vi "Day 4 - Part two.vi"() -> ()   [LabVIEW 2023]
panel:
  out "appended array":string[][](array[string])
  out "sum":i16
  in  "input":string="71-89,66-70\n24-70,23-55\n19-85,18-86\n50-90,50-95\n55-55,56-72\n3-65,5-66\n98-99,66-99\n14-67,14-14\n4-79,78-79\n13-98,10-98\n27-78,77-78\n22-28,22-27\n84-99,98-99\n7-96,99-99\n33-54,34-54\n29-45,44-44\n18-48,57-78\n89-95,89-93\n39-53,63-99\n13-95,94-95\n7-43,7-42\n16-16,16-96\n41-68,68-87\n83-83,73-82\n65-95,64-71\n5-98,5-95\n51-54,50-99\n33-39,36-74\n9-73,10-86\n20-31,21-59\n12-27,11-12\n10-96,7-11\n55-71,70-77\n13-97,3-14\n5-99,5-5\n25-98,25-98\n81-94,81-94\n26-42,49-74\n77-98,31-77\n8-77,6-8\n48-61,60-61\n11-14,13-52\n97-97,1-96\n48-83,48-82\n44-76,75-93\n21-89,20-89\n10-68,9-91\n2-79,78-80\n10-97,96-97\n9-11,10-76\n44-45,45-97\n34-57,27-56\n12-88,12-87\n16-77,16-16\n74-84,14-75\n22-36,21-85\n15-70,9-70\n81-97,3-81\n24-97,23-79\n8-54,54-55\n18-73,17-74\n22-79,39-79\n2-3,2-73\n1-90,1-90\n59-96,19-96\n31-71,31-31\n62-63,63-64\n15-92,91-93\n73-74,18-78\n64-96,65-96\n5-7,6-64\n96-98,2-97\n62-81,51-62\n38-40,33-39\n26-96,21-95\n31-86,30-87\n11-94,2-11\n3-53,30-52\n28-77,27-98\n17-48,44-69\n9-89,1-89\n42-97,42-99\n1-3,2-93\n16-17,17-21\n95-99,14-96\n51-99,52-57\n28-35,28-35\n30-90,76-91\n4-97,4-4\n78-92,14-57\n74-97,75-97\n15-94,14-94\n29-68,29-69\n1-95,2-30\n6-84,98-99\n12-72,71-72\n5-6,5-30\n19-63,63-72\n4-99,3-99\n5-61,62-62\n35-55,34-56\n11-58,75-87\n4-98,3-98\n33-34,34-77\n56-94,55-95\n8-78,99-99\n19-20,19-90\n58-90,43-57\n87-94,22-84\n20-50,49-60\n14-15,16-90\n7-93,7-89\n7-97,7-7\n4-88,4-89\n35-49,48-56\n53-85,55-94\n5-66,4-6\n17-78,19-78\n6-28,28-66\n55-88,91-98\n21-22,21-94\n18-42,17-42\n4-98,6-98\n10-96,97-99\n25-89,89-93\n5-98,1-5\n62-77,63-73\n12-37,11-38\n17-29,17-29\n51-62,45-61\n86-87,44-86\n33-88,22-33\n89-89,14-88\n89-89,53-81\n61-63,59-64\n56-75,55-75\n21-93,20-90\n81-82,81-82\n8-86,87-96\n3-99,4-98\n30-30,30-33\n3-59,2-59\n58-72,7-70\n45-67,16-45\n14-37,13-13\n29-47,14-46\n2-85,1-3\n61-98,81-86\n16-35,17-80\n4-92,4-92\n10-38,11-97\n92-93,20-93\n40-53,41-53\n28-84,3-35\n11-96,6-36\n57-81,57-82\n77-86,6-77\n4-67,4-67\n55-57,56-76\n26-27,27-45\n44-47,44-46\n7-98,6-99\n10-51,9-87\n10-41,10-10\n7-37,7-90\n55-97,54-54\n21-97,20-64\n64-85,44-53\n31-47,46-59\n67-78,68-95\n27-95,26-66\n11-82,54-83\n52-75,24-67\n13-84,6-84\n37-48,33-41\n27-28,28-57\n23-95,86-95\n8-8,8-28\n27-74,26-28\n56-82,42-56\n9-59,14-59\n26-62,61-94\n1-2,1-88\n83-92,97-98\n13-91,13-30\n42-96,95-96\n43-97,34-97\n45-82,15-69\n90-90,65-91\n25-89,26-26\n16-36,15-15\n14-80,79-79\n49-72,49-50\n19-47,18-88\n7-46,7-23\n14-24,24-80\n2-2,3-98\n2-99,2-99\n14-44,14-14\n25-27,6-27\n28-96,27-97\n24-75,23-81\n10-74,13-75\n61-62,13-62\n94-95,96-98\n22-24,22-82\n10-10,10-81\n37-77,76-77\n10-32,18-32\n8-79,7-7\n45-46,45-77\n16-21,16-20\n8-45,44-57\n19-61,18-61\n9-67,9-66\n4-86,1-86\n49-63,48-63\n39-83,23-82\n3-67,18-67\n74-84,83-83\n32-77,33-77\n14-55,5-49\n59-73,26-73\n15-55,16-83\n19-19,20-43\n59-60,32-60\n30-58,33-39\n9-76,9-76\n67-81,21-68\n37-37,28-38\n64-75,63-84\n5-91,11-88\n41-95,37-96\n46-76,76-87\n39-82,40-82\n92-95,2-93\n92-93,1-93\n4-97,4-98\n31-75,30-75\n97-98,2-97\n78-78,40-77\n36-36,36-41\n5-93,4-94\n29-92,29-92\n41-88,42-92\n9-50,47-51\n16-87,16-16\n18-63,62-63\n89-92,90-95\n80-81,16-81\n3-34,4-34\n13-97,96-98\n1-93,92-94\n34-88,35-87\n97-98,43-97\n41-76,42-69\n28-33,27-46\n1-35,3-99\n9-95,10-94\n15-99,15-92\n93-94,1-94\n42-92,43-94\n91-98,71-90\n19-50,47-50\n24-91,94-99\n10-98,11-98\n42-87,86-86\n18-92,48-92\n52-52,5-51\n73-80,32-74\n43-46,39-50\n41-45,40-44\n48-86,49-68\n55-67,56-67\n34-94,34-34\n16-72,17-71\n27-75,33-75\n3-34,33-34\n27-70,70-71\n85-97,31-84\n46-46,21-47\n1-98,97-99\n15-90,5-90\n10-63,10-62\n3-4,5-77\n18-41,23-62\n32-80,33-79\n17-17,17-89\n63-83,15-83\n5-82,5-82\n51-60,51-82\n1-82,1-82\n9-14,13-97\n10-99,13-99\n70-89,88-97\n84-89,83-90\n80-86,25-85\n29-88,29-89\n5-68,10-68\n95-96,47-78\n26-95,26-96\n1-2,2-87\n32-57,21-58\n3-99,2-3\n93-93,50-94\n62-96,62-89\n52-82,52-81\n27-82,27-27\n39-79,38-39\n17-97,16-97\n2-90,1-91\n43-48,43-52\n5-25,9-25\n4-95,4-5\n14-59,13-59\n44-81,43-43\n95-96,20-96\n13-14,11-14\n26-91,20-91\n23-64,64-64\n20-95,21-21\n4-85,4-84\n17-60,15-60\n79-80,66-79\n78-95,78-90\n34-38,33-38\n41-49,48-49\n4-44,3-44\n68-68,10-69\n4-83,82-84\n86-88,12-87\n2-37,36-75\n7-57,58-81\n11-13,12-99\n6-93,5-90\n28-84,29-56\n6-93,3-3\n35-63,36-72\n7-7,7-55\n27-44,19-44\n41-86,30-80\n1-82,2-81\n1-3,3-92\n2-10,4-52\n12-98,8-11\n5-10,4-27\n47-79,46-46\n47-96,97-98\n74-82,74-75\n36-95,11-35\n10-18,17-24\n32-34,33-48\n9-83,9-83\n7-92,19-92\n12-92,12-86\n7-81,7-82\n24-74,38-73\n19-26,1-26\n5-11,4-11\n13-82,14-81\n33-98,32-33\n30-97,96-96\n28-79,79-81\n60-91,59-86\n50-94,50-94\n74-98,57-73\n5-85,4-37\n4-90,3-71\n22-76,22-76\n48-51,51-65\n4-56,5-55\n2-72,46-71\n18-99,17-93\n98-99,3-98\n14-66,14-79\n12-73,13-72\n16-19,2-17\n2-98,3-98\n65-97,65-96\n9-38,37-38\n9-55,10-95\n49-65,26-66\n7-85,7-86\n18-20,7-19\n33-73,33-73\n18-89,35-56\n1-81,1-71\n18-65,17-65\n84-97,59-94\n10-73,72-73\n2-90,3-66\n13-41,4-29\n1-99,86-99\n20-96,19-68\n84-85,83-85\n27-92,27-92\n20-70,19-19\n11-96,12-97\n35-86,34-36\n8-9,8-22\n9-72,8-72\n5-89,5-57\n46-58,57-59\n41-41,42-75\n32-84,31-88\n39-91,90-91\n6-39,5-60\n51-69,70-83\n5-78,32-75\n8-92,8-8\n2-3,4-81\n70-95,14-95\n10-15,16-72\n26-64,29-63\n26-83,27-82\n48-93,44-47\n76-90,76-91\n73-99,74-74\n9-71,8-41\n13-13,13-91\n32-81,32-80\n9-95,9-95\n97-99,84-96\n90-91,52-90\n2-96,2-97\n73-99,2-97\n6-33,7-27\n9-67,10-67\n47-48,47-59\n3-87,87-99\n35-53,49-64\n40-98,41-93\n52-86,33-85\n23-55,89-91\n29-90,91-96\n5-69,5-69\n27-29,28-68\n14-33,81-88\n2-79,79-98\n34-92,93-94\n1-66,2-66\n8-96,7-97\n12-96,97-98\n78-92,10-88\n86-86,2-87\n11-65,2-64\n19-42,20-41\n2-34,34-93\n36-42,36-43\n10-86,11-78\n2-22,2-71\n8-20,19-95\n5-99,6-89\n6-18,6-6\n3-6,10-81\n69-71,69-69\n52-62,52-62\n79-98,79-98\n49-93,49-70\n10-97,10-97\n23-32,12-24\n7-8,8-94\n37-98,97-97\n2-80,2-79\n33-82,18-98\n53-65,54-90\n68-95,68-96\n7-8,7-14\n24-92,24-91\n31-36,32-48\n13-83,13-82\n23-54,53-53\n43-52,10-43\n24-66,23-94\n19-51,49-68\n66-72,39-66\n23-67,66-67\n34-80,48-79\n83-96,33-82\n79-90,33-95\n10-96,9-78\n12-97,96-99\n10-44,13-96\n2-94,93-93\n5-94,5-94\n71-95,74-97\n60-95,59-96\n86-95,14-86\n4-99,4-54\n12-47,13-13\n23-34,22-34\n49-96,49-86\n37-59,37-59\n1-4,3-94\n9-91,9-91\n57-99,45-57\n8-13,11-13\n11-85,84-85\n47-92,48-92\n4-89,5-89\n4-30,29-31\n10-65,9-64\n60-63,62-92\n43-78,23-42\n16-46,45-47\n26-95,95-96\n63-63,12-64\n21-47,20-47\n14-97,20-98\n6-90,6-86\n71-83,13-72\n64-91,83-90\n5-8,5-7\n42-84,41-98\n30-59,29-60\n6-92,5-95\n5-39,4-40\n71-85,16-70\n2-92,2-91\n8-91,20-91\n72-99,3-71\n31-82,97-98\n78-89,77-90\n48-89,47-89\n63-64,64-64\n24-74,73-88\n1-97,98-99\n73-82,72-82\n13-29,30-98\n11-41,11-12\n36-53,33-52\n46-90,66-89\n4-7,8-87\n5-45,46-91\n11-39,12-78\n42-93,41-85\n40-91,40-91\n23-27,23-51\n3-20,3-21\n64-91,48-91\n57-62,86-91\n5-21,22-89\n45-86,43-86\n94-97,54-93\n13-61,60-60\n25-98,19-97\n34-37,36-37\n97-98,16-96\n4-96,24-95\n2-55,1-92\n62-65,61-73\n21-52,20-21\n43-85,85-86\n2-95,2-95\n10-92,9-92\n8-99,9-98\n23-76,77-90\n18-18,1-19\n47-59,46-60\n78-84,77-81\n23-98,24-96\n2-61,1-60\n37-57,37-56\n58-74,58-58\n28-68,27-67\n16-84,17-84\n1-36,1-36\n62-63,14-63\n22-99,23-98\n1-86,85-86\n47-98,46-82\n4-72,5-72\n41-82,41-79\n64-95,64-93\n14-98,13-95\n38-83,35-83\n69-70,26-69\n1-99,2-72\n18-20,19-82\n12-34,11-34\n68-94,95-95\n59-89,89-90\n71-73,73-75\n58-78,18-92\n32-73,21-33\n31-91,90-91\n28-90,89-90\n54-56,77-94\n15-15,16-79\n57-88,24-57\n8-96,7-82\n5-50,5-50\n34-53,54-54\n75-75,62-76\n1-99,2-49\n4-4,3-61\n16-51,17-52\n19-99,4-44\n20-75,19-20\n36-57,21-35\n9-99,9-96\n15-61,38-61\n98-98,99-99\n2-94,13-94\n15-52,16-51\n10-98,12-98\n1-44,1-89\n4-97,3-97\n20-36,21-36\n28-29,29-79\n1-76,1-74\n69-69,69-94\n47-47,47-59\n15-22,21-91\n57-57,57-80\n11-11,11-35\n6-59,58-64\n15-70,15-71\n52-79,51-64\n60-65,55-64\n20-55,21-54\n26-75,99-99\n82-82,48-83\n4-81,82-82\n12-45,44-45\n3-80,2-81\n11-98,1-12\n21-41,35-41\n41-93,40-40\n87-99,1-87\n11-82,11-82\n5-86,4-8\n93-93,5-77\n11-94,1-10\n38-58,39-58\n63-64,35-62\n2-98,3-56\n9-75,76-77\n52-85,52-85\n32-36,32-36\n44-87,43-84\n4-85,84-85\n85-96,12-95\n2-66,26-66\n23-33,8-22\n16-92,15-80\n72-86,72-86\n8-42,7-7\n14-53,15-53\n4-78,8-78\n41-98,27-99\n33-40,4-39\n12-78,13-89\n9-93,10-93\n91-98,92-98\n30-90,29-69\n33-50,2-34\n22-89,23-89\n28-93,93-99\n5-45,4-45\n12-85,86-91\n52-99,52-99\n14-81,82-92\n3-98,4-69\n64-92,8-99\n1-90,5-90\n38-77,26-91\n49-65,35-42\n3-94,4-74\n4-58,4-4\n2-96,95-97\n2-99,3-98\n21-94,20-95\n11-76,12-75\n2-96,92-95\n44-76,41-76\n5-93,6-92\n85-90,20-89\n5-13,12-28\n97-97,96-98\n34-87,34-88\n14-27,14-35\n79-80,17-79\n6-23,22-52\n5-78,72-83\n25-80,26-46\n51-79,90-97\n28-80,77-80\n87-90,24-89\n89-90,71-90\n16-96,16-23\n32-86,31-31\n9-83,9-10\n46-53,52-53\n28-93,92-93\n41-50,40-48\n48-64,47-71\n5-23,3-6\n44-85,7-85\n30-57,29-58\n5-95,8-90\n6-95,12-95\n29-95,29-99\n15-44,14-14\n28-94,28-97\n8-8,7-8\n35-35,36-67\n35-88,71-93\n89-90,27-90\n89-91,30-90\n57-82,56-57\n24-74,19-74\n2-95,2-95\n55-91,54-91\n86-89,87-91\n30-81,30-81\n52-77,53-66\n5-91,75-90\n41-77,50-77\n52-73,34-69\n33-37,32-37\n40-71,74-85\n9-34,33-33\n95-95,25-96\n12-50,51-95\n16-65,53-60\n15-75,16-27\n6-33,6-7\n10-30,36-57\n10-60,2-60\n28-58,57-94\n16-62,15-62\n96-98,10-97\n19-28,8-47\n4-94,93-93\n2-96,95-96\n58-60,36-59\n8-62,13-98\n21-96,21-34\n11-50,11-50\n49-93,95-97\n6-76,8-99\n65-99,65-92\n13-66,3-54\n13-95,94-94\n57-96,57-96\n42-85,57-84\n26-81,25-82\n54-98,54-86\n3-84,83-92\n7-72,8-51\n67-83,67-71\n6-34,14-39\n1-47,1-47\n97-97,12-94\n2-89,2-98\n12-16,15-87\n30-59,31-59\n78-82,80-83\n14-69,9-70\n9-97,9-99\n45-68,44-69\n24-51,47-48\n48-48,48-68\n75-77,47-53\n7-73,7-73\n9-72,8-66\n39-70,38-71\n39-69,68-98\n26-94,26-93\n14-63,15-62\n19-61,61-62\n7-15,11-99\n1-73,2-51\n44-90,90-91\n54-97,96-98\n1-93,11-20\n34-70,35-69\n11-11,11-87\n8-73,8-73\n15-23,24-85\n42-57,43-99\n23-29,13-67\n99-99,1-54\n65-66,21-65\n23-38,23-75\n84-94,18-94\n10-63,11-62\n33-35,34-38\n68-70,4-69\n4-8,7-94\n20-95,20-54\n11-99,4-44\n20-97,3-97\n7-85,85-96\n44-85,45-84\n9-17,5-10\n82-97,22-81\n4-98,3-98\n17-80,17-75\n22-49,22-49\n94-99,27-91\n49-91,17-50\n20-30,36-49\n8-84,83-84\n59-91,60-73\n76-93,2-97\n5-48,5-94\n22-67,21-21\n3-4,4-5\n20-95,21-99\n21-86,85-87\n38-44,36-43\n2-90,91-99\n60-67,3-60\n3-58,4-57\n46-84,46-82\n13-13,14-95\n30-74,73-74\n24-34,24-34\n4-98,5-98\n6-7,2-6\n41-98,42-98\n16-58,57-85\n86-90,61-86\n2-85,2-84\n7-90,90-93\n25-65,26-30\n41-69,12-70\n31-88,32-87\n10-87,10-87\n4-29,4-98\n8-40,30-40\n26-82,25-82\n89-90,88-89\n4-13,9-14\n10-65,6-7\n6-13,13-99\n75-79,45-79\n6-98,9-89\n6-55,54-58\n2-78,25-78\n3-98,3-98\n95-95,6-94\n9-78,77-77\n56-57,56-58\n49-87,24-66\n47-47,47-73\n33-35,6-34\n30-80,36-80\n30-30,31-81\n99-99,68-74\n2-99,3-98\n14-92,10-15\n16-31,18-51\n95-97,2-94\n31-31,15-32\n98-99,68-93\n14-71,14-15\n5-39,14-38\n47-54,53-55\n37-64,37-37\n58-78,10-58\n40-88,41-41\n68-99,16-94\n25-25,26-58\n84-87,1-99\n72-87,72-78\n49-81,48-49\n1-99,2-99\n24-91,25-93\n12-81,11-58\n1-16,15-50\n12-26,12-26\n17-80,17-79\n94-96,38-95\n1-84,83-84\n20-82,20-20\n3-86,2-95\n19-98,60-94\n9-45,45-50\n8-57,9-12\n15-18,18-83\n1-1,1-15\n85-96,84-95\n1-40,40-78\n57-58,30-58\n48-90,57-89\n26-51,27-86\n2-86,85-86\n25-78,26-77\n82-99,81-97\n1-14,13-97\n76-96,75-97\n66-94,64-97\n34-60,38-61\n80-95,22-81\n51-80,51-80\n2-78,1-78\n43-46,45-69\n75-85,76-76\n33-65,32-32\n15-96,14-96\n68-86,67-71\n12-26,12-16\n1-51,3-43\n87-88,27-88\n17-99,16-99\n9-36,20-24\n25-32,24-32\n32-32,32-76\n77-92,52-78\n4-79,4-82\n38-61,54-59\n38-99,38-99\n94-98,54-95\n80-96,2-95\n8-97,8-97\n7-28,8-22\n66-82,83-91\n33-48,49-83\n3-3,4-83\n76-90,77-90\n34-62,34-61\n40-87,16-27\n1-98,2-98\n55-96,95-98\n5-99,5-5\n36-97,10-98\n12-94,93-94\n72-78,71-78\n13-18,14-18\n47-76,75-76\n21-96,21-95\n69-96,68-87\n27-64,28-62\n19-40,25-39\n4-59,4-98\n10-66,10-67\n16-82,17-82\n7-99,3-99\n18-30,17-92\n86-99,24-52\n19-77,20-77\n97-97,93-94\n11-33,10-11\n84-96,53-95\n3-85,4-91\n15-52,16-53\n86-90,52-56\n33-76,33-76\n3-98,17-92\n79-79,4-80\n85-85,2-84\n13-94,94-96\n60-84,90-93\n93-97,15-98\n9-54,10-53\n28-59,27-98\n12-85,11-65\n59-67,58-67\n20-50,20-65\n63-65,16-64\n76-96,75-75\n23-91,24-91\n3-99,3-97\n25-48,26-48\n48-48,49-87\n15-96,1-16\n9-79,25-78\n52-61,62-84\n6-85,7-84\n54-77,53-78\n1-99,1-99\n59-96,60-96\n12-45,12-46\n22-87,3-87\n36-98,36-74\n56-56,22-57\n94-95,99-99\n7-92,8-83\n13-94,14-93\n22-90,89-89\n46-94,83-87\n11-76,75-78\n3-94,3-95\n4-14,5-52\n90-92,66-83\n46-61,46-47\n22-23,22-90\n47-47,48-53\n89-91,16-90\n42-93,93-94\n9-61,60-94\n1-1,1-67\n3-38,2-99\n46-98,47-97\n96-97,1-95\n8-54,55-92\n52-72,53-71"
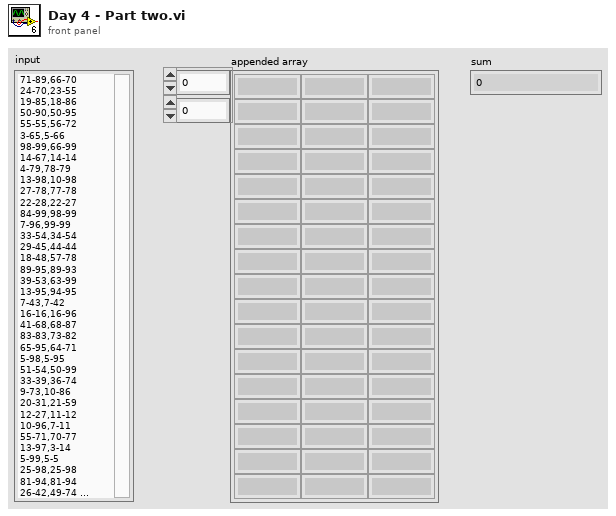
[diagram p1: front panel]
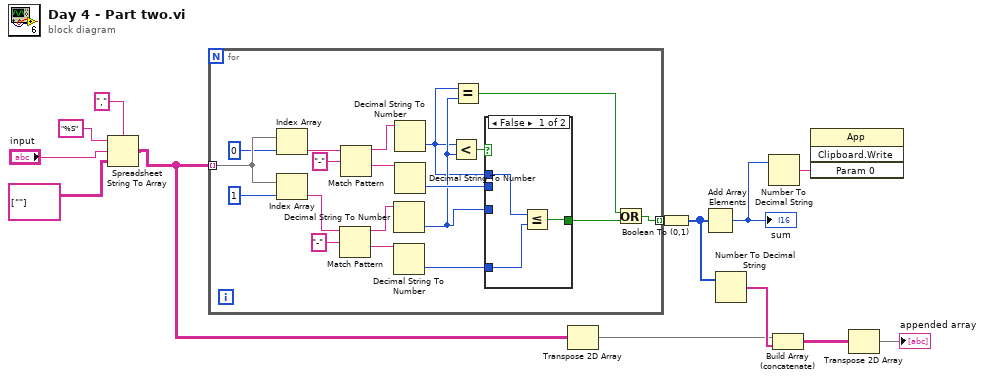
[diagram p0: block diagram]
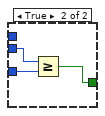
[diagram p2: hidden frame]
diagram:
  n1 = Spreadsheet String To Array(delimiter (Tab)=",", format string="%S", spreadsheet string="input", array type (2D Dbl)=string[][] [[""]]) -> (array=w5:string[][])
  n2 = for {
    tunnel: w5 -> [w32] mode=indexing
    tunnel: [w18] -> w9 mode=indexing
    n3 = Index Array(array=w32, index=0) -> (element=w20:string)
    n4 = Index Array(array=w32, index=1) -> (element=w23:string)
    n5 = Match Pattern(string=w23, regular expression="-") -> (before substring=w25:string, after substring=w26:string)  [unwired: 1 in, 2 out]
    n6 = Match Pattern(string=w20, regular expression="-") -> (before substring=w28:string, after substring=w27:string)  [unwired: 1 in, 2 out]
    n7 = Decimal String To Number(string=w25) -> (number=w16:i32)  [unwired: 2 in, 1 out]
    n8 = Decimal String To Number(string=w26) -> (number=w14:i32)  [unwired: 2 in, 1 out]
    n9 = Decimal String To Number(string=w28) -> (number=w15:i32)  [unwired: 2 in, 1 out]
    n10 = Decimal String To Number(string=w27) -> (number=w21:i32)  [unwired: 2 in, 1 out]
    n11 = Less?(x=w15, y=w16) -> (x < y?=w22:bool)
    n12 = Equal?(x=w15, y=w16) -> (x = y?=w17:bool)
    n13 = case shown="False" w22 {
      tunnel: w21 -> [_ w38]
      tunnel: [w35 w36] -> w19
      tunnel: w16 -> [_ w37]
      tunnel: w15 -> [w34 _]
      tunnel: w14 -> [w33 _]
      frame False {
        n14 = Less Or Equal?(x=w34, y=w33) -> (x <= y?=w35:bool)
      }
      frame True {
        n15 = Greater Or Equal?(x=w38, y=w37) -> (x >= y?=w36:bool)
      }
    }
    n16 = Or(x=w17, y=w19) -> (x .or. y?=w18:bool)
  }
  n17 = Transpose 2D Array(2D array=w5) -> (transposed array=w4:string[][])
  n18 = Boolean To (0,1)(Boolean=w9) -> (0, 1=w8:i16[])
  n19 = Add Array Elements(numeric array=w8) -> (sum=w2:i16)
  "sum" <- w2
  n20 = Number To Decimal String(number=w8) -> (decimal integer string=w7:string[])  [unwired: 1 in]
  n21 = Number To Decimal String(number=w2) -> (decimal integer string=w1:string)  [unwired: 1 in]
  n22 = Build Array (concatenate)(w4, w7) -> (w6:string[][])
  n23 = invoke class="App" method="Clipboard.Write"("Param 0"=w1) -> ()  [unwired: 3 in, 4 out]
  n24 = Transpose 2D Array(2D array=w6) -> (transposed array=→"appended array":string[][])
